vi "INI-FPexample.vi"() -> ()   [LabVIEW 2021]
panel:
  in  "Mode":enum16{"Read", "Write"}(ring)
  in  "outerTab":enum32{"outerP1", "outerP2", "outerP3"}(tab)
  in  "Page1outer":dbl
  in  "innerTab":enum32{"innerP1", "innerP2"}(tab)
  in  "Page1innerB":string
  in  "Page1innerA":string
  in  "innerPage2B":string
  in  "innerPage2A":string
  in  "pag2OuterB":dbl
  in  "pag2OuterA":dbl
  in  "Cluster":T1
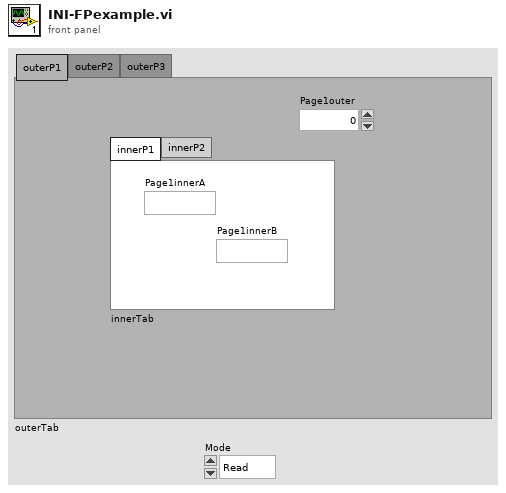
[diagram p1: front panel]
types:
  T1 = cluster{"numInClust":dbl, "stringInCluster":string, "path":path}
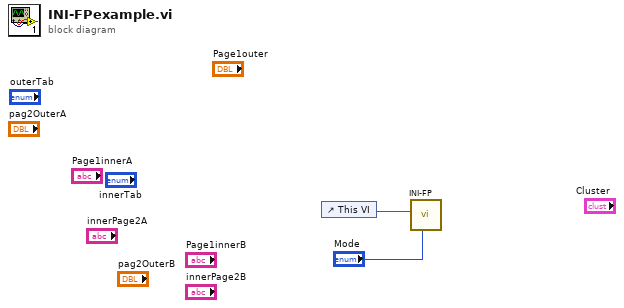
[diagram p0: block diagram]
diagram:
  n1 = control-ref of="This VI"() -> (w2:refnum<vi>)
  n2 = call "INI-FP.vi"("Mode"="Mode", "VIreference"=w2) -> ()  [unwired: 9 in, 1 out]
